vi "Calculate Scaling Info.vi"(9 "DrawAreaSize":T3={"Width"=100, "Height"=100}, 10 "cartesian data":T2, 11 "draw options in":T4={"Background Color"=16777215, "Grid Color"=13816530, "Angle Units"=enum."Radians", "Draw Solid Background"=TRUE, "Draw Grid"=TRUE, "Grid Spacing"=1.0, "AutoScale"=TRUE, "Fit to Radius"=1.0, "data row options"=[]}) -> (3 "scaling info":T1={"pixels per unit"=1.0, "fit radius (units)"=1.0, "center point (pixels)"={"x"=0, "y"=0}})   [LabVIEW 2017, in "NI_Robotics_2D Rangefinder Picture.lvlib"]
uses:
  <vilib>/robotics/Controls/2D Rangefinder/2D Rangefinder Picture/NI_Robotics_2D Rangefinder Picture.lvlib
  <vilib>/robotics/Controls/2D Rangefinder/2D Rangefinder Picture/Draw Options.ctl
  <vilib>/robotics/Controls/Utilities/Angle Units.ctl
  <vilib>/robotics/Controls/2D Rangefinder/2D Rangefinder Picture/Data Row Options.ctl
  <vilib>/Utility/miscctls.llb/LVBoundsTypeDef.ctl
  <vilib>/robotics/Controls/2D Rangefinder/2D Rangefinder Picture/Cartesian Data.ctl
  <vilib>/robotics/Controls/2D Rangefinder/2D Rangefinder Picture/Scaling Info.ctl
  <vilib>/robotics/Controls/Utilities/NI_Robotics_Control Utilities.lvlib
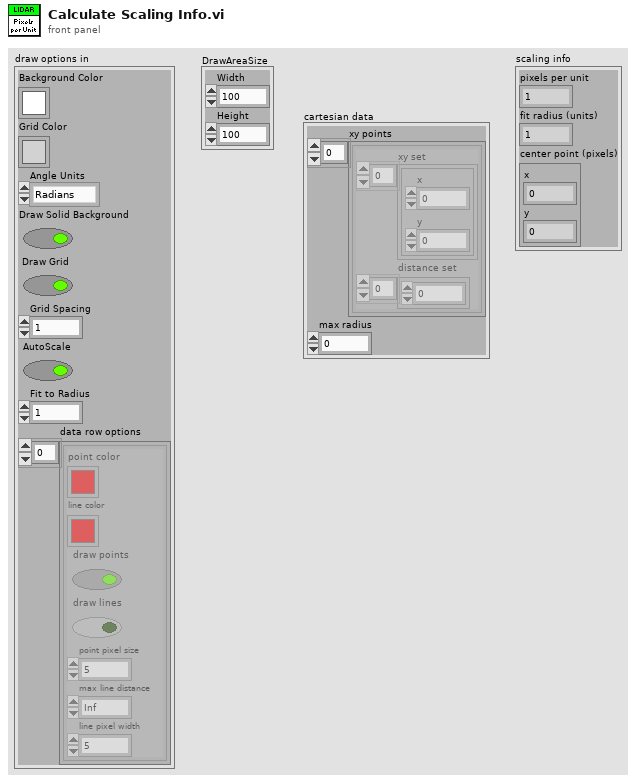
[diagram p1: front panel]
types:
  T1 = typedef "NI_Robotics_2D Rangefinder Picture.lvlib/Scaling Info.ctl" = cluster{"pixels per unit":dbl, "fit radius (units)":dbl, "center point (pixels)":cluster{"x":i16, "y":i16}}
  T2 = typedef "NI_Robotics_2D Rangefinder Picture.lvlib/Cartesian Data.ctl" = cluster{"xy points":cluster{"xy set":cluster{"x":dbl, "y":dbl}[], "distance set":dbl[]}[], "max radius":dbl}
  T3 = typedef "LVBoundsTypeDef.ctl" = cluster{"Width":u32, "Height":u32}
  T4 = typedef "NI_Robotics_2D Rangefinder Picture.lvlib/Draw Options.ctl" = cluster{"Background Color":u32, "Grid Color":u32, "Angle Units":T5, "Draw Solid Background":bool, "Draw Grid":bool, "Grid Spacing":dbl, "AutoScale":bool, "Fit to Radius":dbl, "data row options":T6[]}
  T5 = typedef "NI_Robotics_Control Utilities.lvlib/Angle Units.ctl" = enum16{"Radians", "Degrees"}
  T6 = typedef "NI_Robotics_2D Rangefinder Picture.lvlib/Data Row Options.ctl" = cluster{"point color":u32, "line color":u32, "draw points":bool, "draw lines":bool, "point pixel size":u16, "max line distance":dbl, "line pixel width":u16}
  T7 = cluster{"xy set":cluster{"x":dbl, "y":dbl}[], "distance set":dbl[]}[]
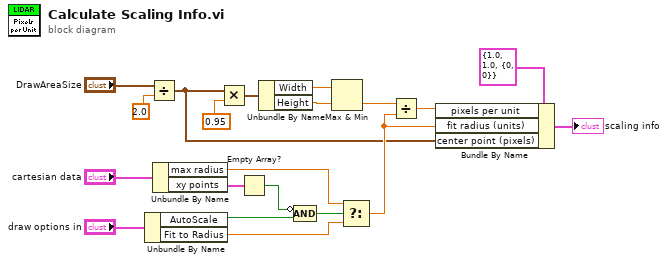
[diagram p0: block diagram]
diagram:
  n1 = Unbundle By Name("draw options in") -> ("AutoScale"=w4:bool, "Fit to Radius"=w9:dbl)
  n2 = Divide(x="DrawAreaSize", y=2.0) -> (x/y=w7:cluster{"Width":dbl, "Height":dbl})
  n3 = Unbundle By Name("cartesian data") -> ("max radius"=w10:dbl, "xy points"=w1:T7)
  n4 = Multiply(x=w7, y=0.95) -> (x*y=w6:cluster{"Width":dbl, "Height":dbl})
  n5 = Empty Array?(array=w1) -> (empty?=w2:bool)
  n6 = Unbundle By Name(w6) -> ("Width"=w13:dbl, "Height"=w14:dbl)
  n7 = Compound Arithmetic op=AND(invert w2, w4) -> (w3:bool)
  n8 = Max & Min(x=w13, y=w14) -> (min(x,y)=w12:dbl)  [unwired: 1 out]
  n9 = Select(t=w10, s=w3, f=w9) -> (s? t:f=w8:dbl)
  n10 = Divide(x=w12, y=w8) -> (x/y=w16:dbl)
  n11 = Bundle By Name(cluster=T1 {"pixels per unit"=1.0, "fit radius (units)"=1.0, "center point (pixels)"={"x"=0, "y"=0}} ("scaling info"), "pixels per unit"=w16, "fit radius (units)"=w8, "center point (pixels)"=w7) -> (→"scaling info":T1)
